vi "NML Oscilloscope.vi"(3 "Range Max":dbl=10.0 min=0.0 max=10.0 format="%.3f", 5 "LEVEL":sgl(knob) scale=-10.0..10.0 scale format="%.2f", 6 "Time Between\nSamples (msec)":dbl=0.1 min=0.001 step=0.001 format="%.3f", 7 "Chan #":i16(slide) min=0 max=7 step=1 scale=0.0..7.0, 8 "Number of Samples":i32=1024) -> (1 "WAVEFORM":T1(graph), 2 "WAVEFORM SAMPLES":dbl[](array[numeric]) format="%.4f")   [LabVIEW 2020]
doc: "This VI is an oscilloscope. It sets up the data acquistion then takes the desired number of samples from the selected channel. The collected samples are scaled and plotted.\nScott Hannahs, FBNML, Jan 1992"
uses:
  <vilib>/Utility/error.llb/DialogType.ctl
  <vilib>/_DAQmxBase/Internals/DAQmxBase Create Channel (AI-Voltage-Basic).vi
  <vilib>/_DAQmxBase/Internals/DAQmxBase Timing (Sample Clock).vi
  <vilib>/_DAQmxBase/Internals/DAQmxBase Start Trigger (Analog Edge).vi
  <vilib>/_DAQmxBase/Internals/DAQmxBase Read (Analog 2D DBL NChan NSamp).vi
  <vilib>/Analysis/NI_AALBase.lvlib
panel:
  in  "Slope":i32(ring)=10280 items=["Rising"=10280, "Falling"=10171]
  in  "Range Min":dbl=-10.0 min=-10.0 max=0.0 format="%.3f"
  in  "Filename":string="Test"
  out "Std. Dev.":dbl format="%.4e"
  out "Average":dbl format="%.4e"
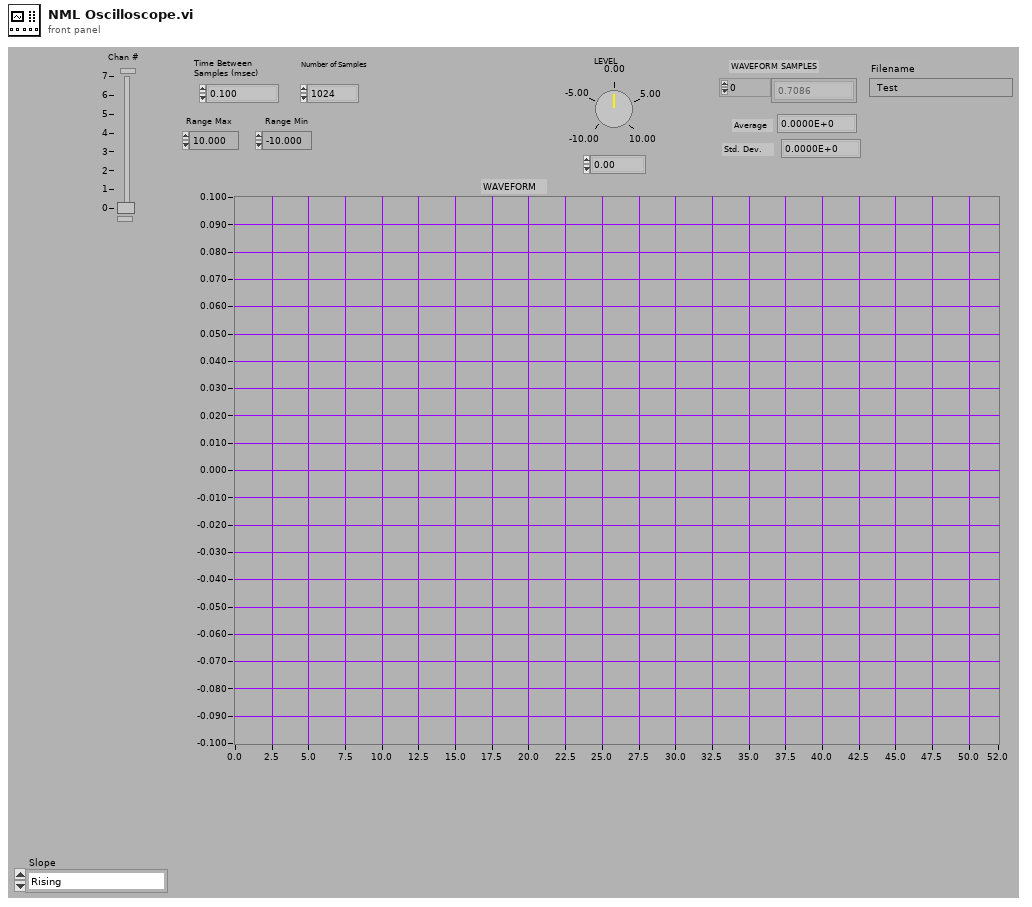
[diagram p1: front panel]
types:
  T1 = cluster{dbl, "Time Between\nSamples (msec)":dbl, dbl[]}
  T2 = typedef "DialogType.ctl" = u16
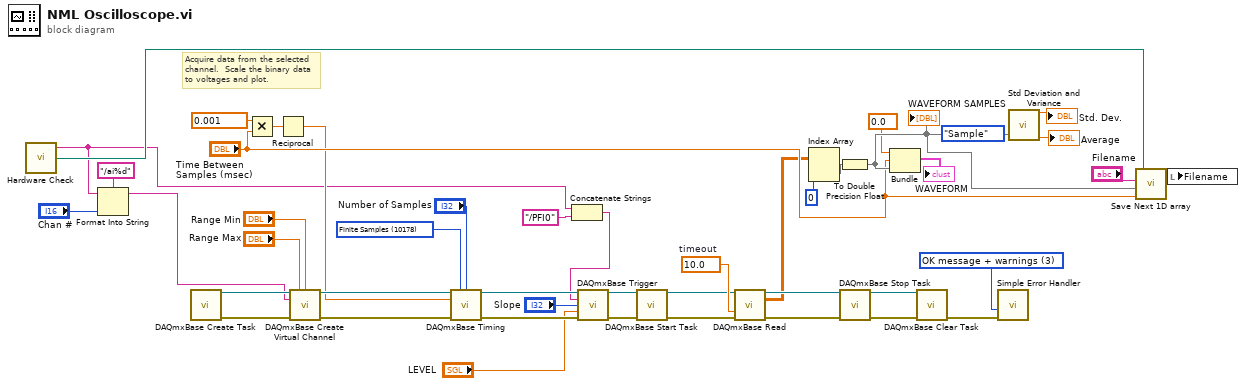
[diagram p0: block diagram]
diagram:
  w20 = T2 3 items=["no dialog", "OK message", "continue or stop message", "OK message + warnings", "continue/stop + warnings"] ("type of dialog (OK msg:1)")
  w24 = 10.0  # timeout
  w31 = 10178 items=["Finite Samples"=10178, "Continuous Samples"=10123] ("sample mode")
  # "Acquire data from the selected\nchannel.  Scale the binary data\nto voltages and plot."
  n1 = call "Hardware Check.vi"() -> ("Data Acq Device"=w1:string, "Data Directory Path"=w40:path)  [unwired: 1 in, 1 out]
  n2 = Format Into String(format string="/ai%d", initial string=w1, "Chan #") -> (resulting string=w5:string)  [unwired: 1 in, 1 out]
  n3 = call <vilib>:"DAQmxBase Create Task.vi"() -> ("task out"=w30:refnum<k21>, "error out"=w13:errorcluster)  [unwired: 14 in]
  n4 = Multiply(x=0.001, y="Time Between\nSamples (msec)") -> (x*y=w44:dbl)
  n5 = Reciprocal(x=w44) -> (1/x=w9:dbl)
  n6 = call-poly <vilib>:"DAQmxBase Create Virtual Channel.vi"("task in"=w30, "maximum value"="Range Max", "minimum value"="Range Min", "physical channels"=w5, "error in"=w13) -> ("task out"=w29:refnum<k21>, "error out"=w14:errorcluster)  [unwired: 9 in]
  n7 = call-poly <vilib>:"DAQmxBase Timing.vi"("task/channels in"=w29, "sample mode"=w31, "samples per channel"="Number of Samples", "rate"=w9, "error in"=w14) -> ("task out"=w26:refnum<k21>, "error out"=w27:errorcluster)  [unwired: 9 in]
  n8 = Concatenate Strings(w1, "/PFI0" ("source")) -> (w2:string)
  n9 = call-poly <vilib>:"DAQmxBase Trigger.vi"("task/channels in"=w26, "source"=w2, "slope"="Slope", "level"="LEVEL", "error in"=w27) -> ("task out"=w25:refnum<k21>, "error out"=w19:errorcluster)  [unwired: 9 in]
  n10 = call <vilib>:"DAQmxBase Start Task.vi"("task/channels in"=w25, "error in"=w19) -> ("task out"=w23:refnum<k21>, "error out"=w15:errorcluster)  [unwired: 12 in]
  n11 = call-poly <vilib>:"DAQmxBase Read.vi"("task/channels in"=w23, "timeout"=w24, "error in"=w15) -> ("task out"=w21:refnum<k21>, "data"=w12:dbl[][], "error out"=w16:errorcluster)  [unwired: 10 in]
  n12 = Index Array(array=w12, index (col)=0) -> (element=w34:dbl[])  [unwired: 1 in]
  n13 = To Double Precision Float(number=w34) -> (double precision float=w43:dbl[])
  "WAVEFORM SAMPLES" <- w43
  n14 = call <vilib>:"DAQmxBase Stop Task.vi"("task/channels in"=w21, "error in"=w16) -> ("task out"=w22:refnum<k21>, "error out"=w17:errorcluster)  [unwired: 12 in]
  n15 = Bundle(0.0, "Time Between\nSamples (msec)"="Time Between\nSamples (msec)", w43) -> (→"WAVEFORM":T1)  [unwired: 1 in]
  n16 = call <vilib>:"DAQmxBase Clear Task.vi"("task in"=w22, "error in"=w17) -> ("error out"=w18:errorcluster)  [unwired: 13 in]
  n17 = call <vilib>:"Simple Error Handler.vi"("type of dialog (OK msg:1)"=w20, "error in (no error)"=w18) -> ()  [unwired: 3 in, 5 out]
  n18 = call <vilib>:"Std Deviation and Variance.vi"("X"=w43, "Weighting (Sample)"=enum16{"Sample", "Population"}."Sample") -> ("mean"=→"Average":dbl, "standard deviation"=→"Std. Dev.":dbl)  [unwired: 1 out]
  n19 = call "Save Next 1D array.vi"("ÆT"="Time Between\nSamples (msec)", "Data"=w43, "File Name"="Filename", "Dir Path"=w40) -> ("New File Name"=w39:string)  [unwired: 1 in]
  n20 = local write "Filename"(w39) -> ()
